vi "RSZVB Set Port Configuration.vi"(5 "Port Group B (0)":i32, 6 "Port Group D (0)":i32, 7 "Port Group C (0)":i32, 8 "error in (no error)":errorcluster {"code" format="%.0x"}, 9 "Port Group A (0)":i32, 10 "Channel (1)":i32=1, 11 "VISA session":refnum<visa-resource-name>) -> (0 "error out":errorcluster {"code" format="%.0x"}, 3 "dup VISA session":refnum<visa-resource-name>)   [LabVIEW 2011]
doc: "This VI configures the internal signal paths of the multiport test set R&S ZV-Z83 for channel no. <Ch>. \n\nRemote-control command(s):\nROUTe<Ch>:PORTs"
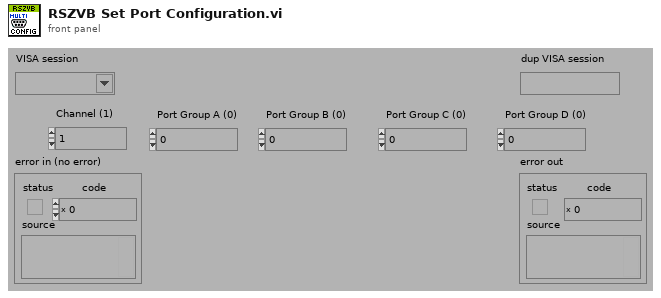
[diagram p1: front panel]
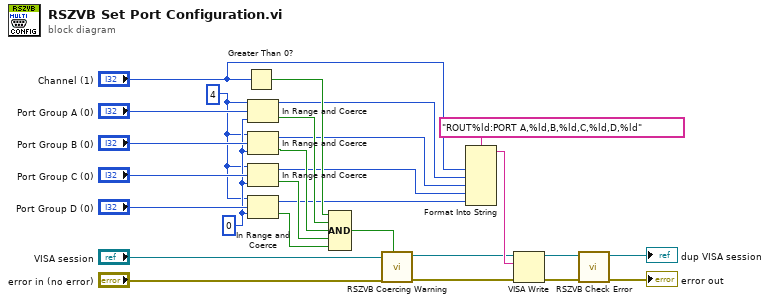
[diagram p0: block diagram]
diagram:
  w9 = 4
  w16 = 0
  n1 = Greater Than 0?(x="Channel (1)") -> (x > 0?=w15:bool)
  n2 = In Range and Coerce(upper limit=w9, x="Port Group A (0)", lower limit=w16) -> (In Range?=w14:bool)  [unwired: 1 out]
  n3 = In Range and Coerce(upper limit=w9, x="Port Group B (0)", lower limit=w16) -> (coerced(x)=w8:i32, In Range?=w13:bool)
  n4 = In Range and Coerce(upper limit=w9, x="Port Group C (0)", lower limit=w16) -> (coerced(x)=w7:i32, In Range?=w12:bool)
  n5 = In Range and Coerce(upper limit=w9, x="Port Group D (0)", lower limit=w16) -> (coerced(x)=w6:i32, In Range?=w11:bool)
  n6 = Compound Arithmetic op=AND(w15, w14, w13, w12, w11) -> (w5:bool)
  n7 = call "RSZVB Coercing Warning.vi"("In Range?"=w5, "error in (no error)"="error in (no error)", "VISA session"="VISA session") -> ("error out"=w25:errorcluster, "dup VISA session"=w24:refnum<visa-resource-name>)  [unwired: 7 in]
  n8 = Format Into String(format string="ROUT%ld:PORT A,%ld,B,%ld,C,%ld,D,%ld", "Channel (1)", w9, w8, w7, w6) -> (resulting string=w26:string)  [unwired: 2 in, 1 out]
  n9 = VISA Write(VISA resource name=w24, write buffer=w26, error in (no error)=w25) -> (VISA resource name out=w4:refnum<visa-resource-name>, error out=w3:errorcluster)  [unwired: 1 out]
  n10 = call "RSZVB Check Error.vi"("error in (no error)"=w3, "VISA session"=w4) -> ("error out"=→"error out":errorcluster, "dup VISA session"=→"dup VISA session":refnum<visa-resource-name>)  [unwired: 8 in]
